vi "writeToXML.vi"(8 "error in (no error)":errorcluster, 10 "ClassLabel":string, 11 "AzElTarget in":refnum<class "AzElTarget.lvclass">) -> (0 "error out":errorcluster, 2 "XMLout":string, 3 "AzElTarget out":refnum<class "AzElTarget.lvclass">)   [LabVIEW 2022 SP3, in "TCSDataDefinitions.lvlib" / "TCSCommand.lvlib" / "TargetConfiguration.lvlib" / "Target.lvlib" / "FixedTarget.lvlib" / "AzElTarget.lvclass"]
uses:
  AzElTarget.lvclass
  AzElTarget.lvclass/AzElTarget.ctl
  FixedTarget/FixedTarget.lvclass
  AzElParameters/AzElParameters.lvclass
  <userlib>/Common/XML/XMLGenerator/XMLGenerator.lvclass
  <userlib>/Common/XML/XMLAttributeGenerator/XMLAttributeGenerator.lvclass
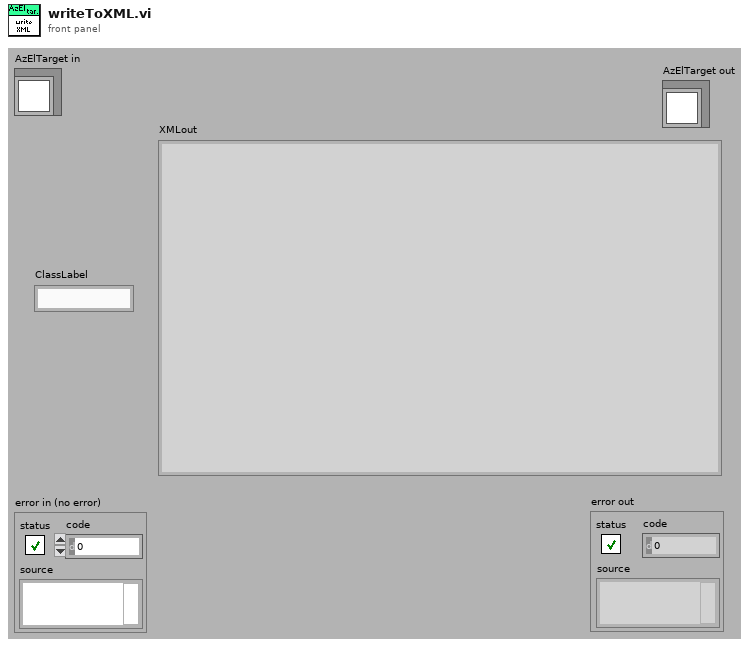
[diagram p1: front panel]
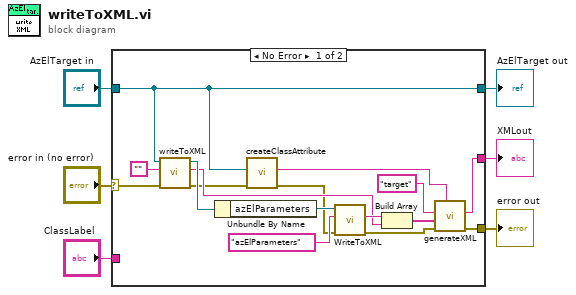
[diagram p0: block diagram]
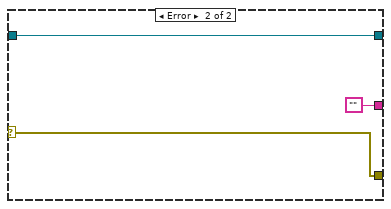
[diagram p2: hidden frame]
diagram:
  n1 = case shown="No Error" "error in (no error)" {
    selector: "error in (no error)" -> [w15 w25]
    tunnel: [w17 w25] -> w5
    tunnel: [w10 w24] -> w3
    tunnel: "AzElTarget in" -> [w10 w24]
    tunnel: [w16 ""] -> w2
    tunnel: "ClassLabel" -> [_ _]
    frame No Error {
      n2 = call-parent "writeToXML.vi"("error in (no error)"=w15, "ClassLabel"="", "FixedTarget in"=w10) -> ("error out"=w9:errorcluster, "XMLout"=w12:string, "FixedTarget out"=w14:refnum<class "AzElTarget.lvclass">)  [unwired: 6 in]
      n3 = Unbundle By Name(w14) -> ("azElParameters"=w22:refnum<class "AzElParameters.lvclass">)
      n4 = call <userlib>:"createClassAttribute.vi"("error in (no error)"=w9, "LVClass In"=w10) -> ("error out"=w7:errorcluster, "AttributeString"=w8:string)  [unwired: 7 in, 1 out]
      n5 = call-dynamic "WriteToXML.vi"("error in (no error)"=w7, "Class Label"="azElParameters", "AzElParameters in"=w22) -> ("error out"=w18:errorcluster, "XML out"=w21:string)  [unwired: 6 in, 1 out]
      n6 = Build Array(w21, w12) -> (w20:string[])
      n7 = call <userlib>:"generateXML.vi"("attributeString"=w8, "error in"=w18, "childrenXML"=w20, "elementName"="target" ("Class Label")) -> ("error out"=w17:errorcluster, "XML out"=w16:string)  [unwired: 5 in, 1 out]
    }
    frame Error {
    }
  }
  "error out" <- w5
  "AzElTarget out" <- w3
  "XMLout" <- w2
